vi "KNR Port 1 DIO.vi"() -> ()   [LabVIEW 2013]
uses:
  <vilib>/rvi/Emulation/niFpgaSctlEmulationGetInTimedLoop.vi
  <vilib>/rvi/Emulation/niFpgaEmulationReportErrorSimple.vi
  <vilib>/rvi/Emulation/niFpgaGetClockAttributes.vi
  <vilib>/rvi/eio/common/nirviEmuTemplateMethod_errors.vi
  <vilib>/rvi/Emulation/niFpgaCriticalErrorInLSC.vi
  <vilib>/eio/EIONode/EIONode.xnode
panel:
  in  "RMC/DIO34":bool
  in  "RMC/DIO3":bool
  in  "RMC/DIO2":bool
  in  "RMC/DIO65":bool
  in  "RMC/DIO1":bool
  in  "RMC/DIO33":bool
  in  "RMC/DIO0":bool
  in  "RMC/DIO32":bool
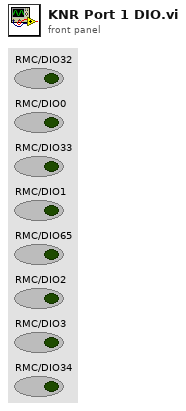
[diagram p1: front panel]
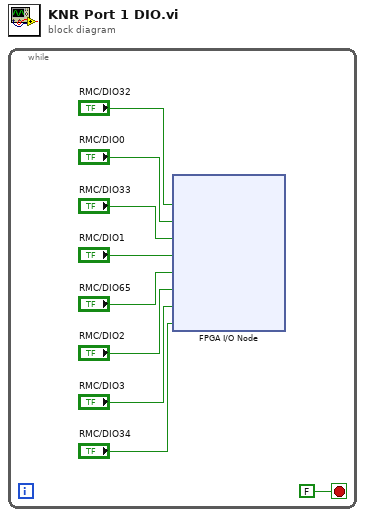
[diagram p0: block diagram]
diagram:
  n1 = while {
    stop <- FALSE stop-if-true
    n2 = xnode "FPGA I/O Node"("RMC/DIO32"="RMC/DIO32", "RMC/DIO0"="RMC/DIO0", "RMC/DIO33"="RMC/DIO33", "RMC/DIO1"="RMC/DIO1", "RMC/DIO65"="RMC/DIO65", "RMC/DIO2"="RMC/DIO2", "RMC/DIO3"="RMC/DIO3", "RMC/DIO34"="RMC/DIO34") -> ()  [unwired: 8 in, 8 out]
  }
